vi "Historical Trend.vi"(8 "error in (no error)":errorcluster, 10 "Subview Stop Event":refnum<user-event>, 11 "Subsystem URL":refnum<k21>="\\\\localhost\\SCADA Server\\Subsystem1") -> ()   [LabVIEW 2024]
doc: "Displays the historical data for the specified subsystems. This VI is a subview of the Detailed View."
uses:
  Controls/Client/Historical Trend - Data.ctl
  Controls/Client/Historical Data.ctl
  Controls/Client/Initialization Status.ctl
  Globals/Global - Client.vi
  Shared/User Event - Stop.lvlib
panel:
  out "error out":errorcluster
  in  "End Time Stamp":timestamp=timestamp(-9593251200 s since 1904-01-01) format="%<%X\n%x>T"
  in  "Start Time Stamp":timestamp=timestamp(-9593251200 s since 1904-01-01) format="%<%X\n%x>T"
  out "Historical Data Graph":T1(graph)
  in  "Stop":bool
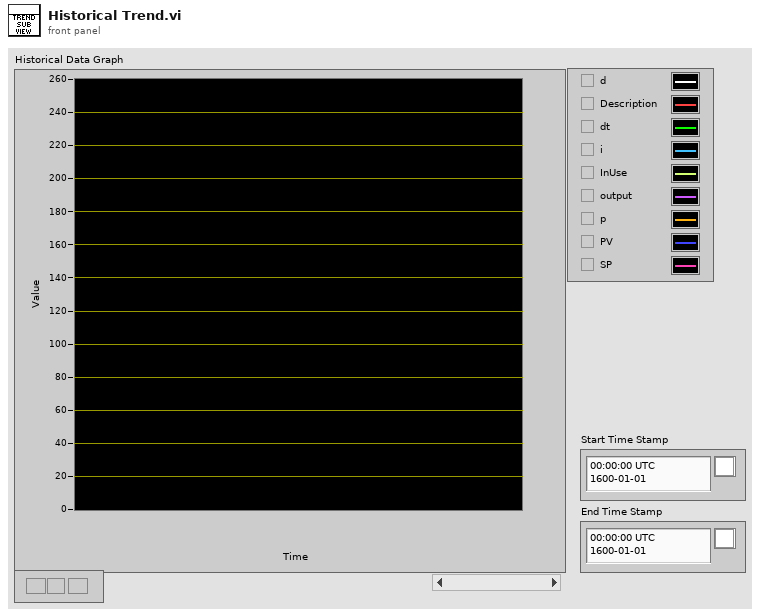
[diagram p1: front panel]
types:
  T1 = cluster{"timestamps":timestamp[], "data":dbl[]}[]
  T2 = typedef "Historical Trend - Data.ctl" = cluster{"Filtered Names":string[], "Variable URLs":refnum<k21>[], "Historical Data":T3[], "Subsystem URL":refnum<k21>, "Subview Stop Event":refnum<user-event>, "Initialization Status":T4}
  T3 = typedef "Historical Data.ctl" = cluster{"timestamps":timestamp[], "data":dbl[]}
  T4 = typedef "Initialization Status.ctl" = enum16{"Initializing", "Initialized"}
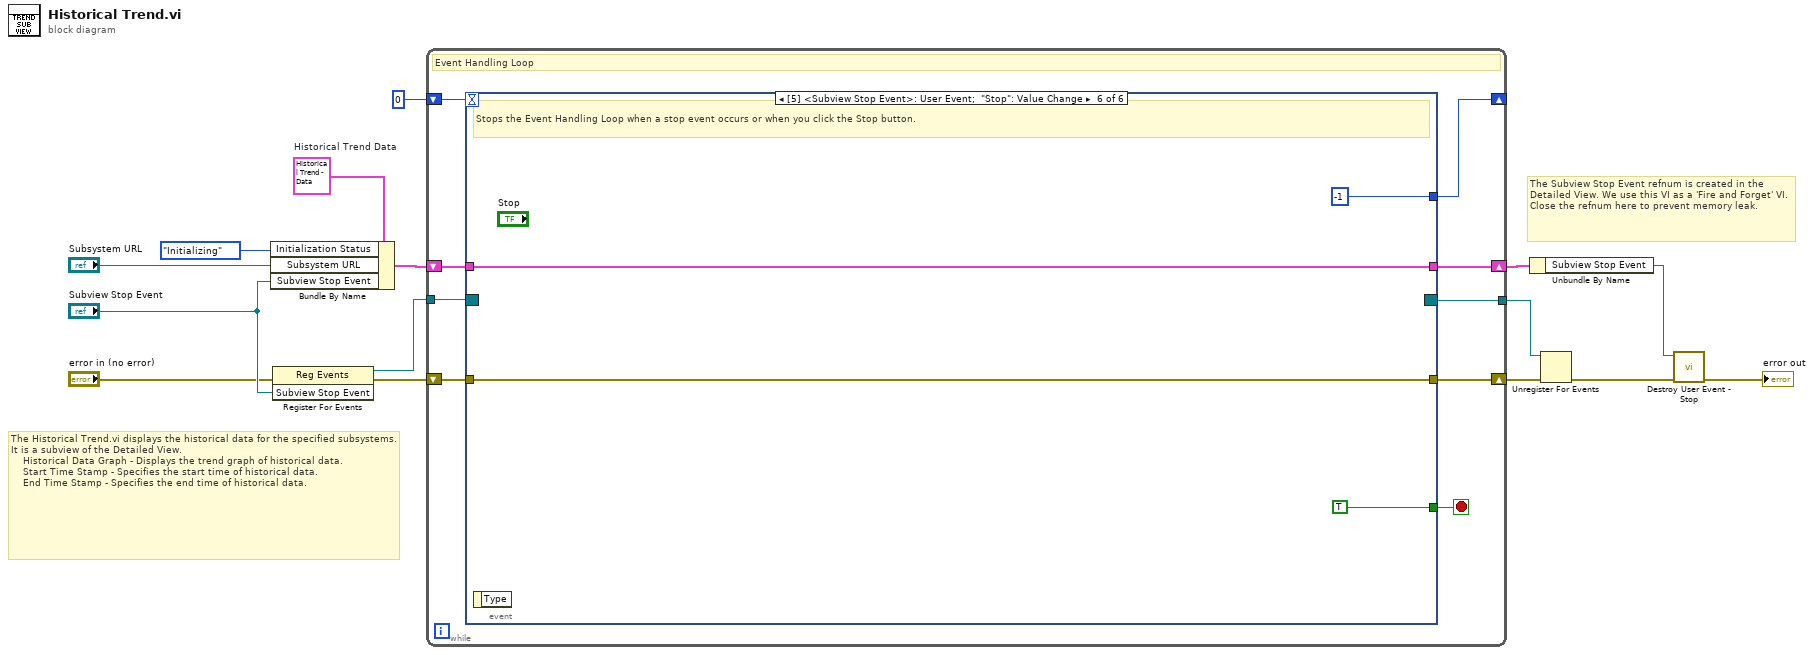
[diagram p0: block diagram]
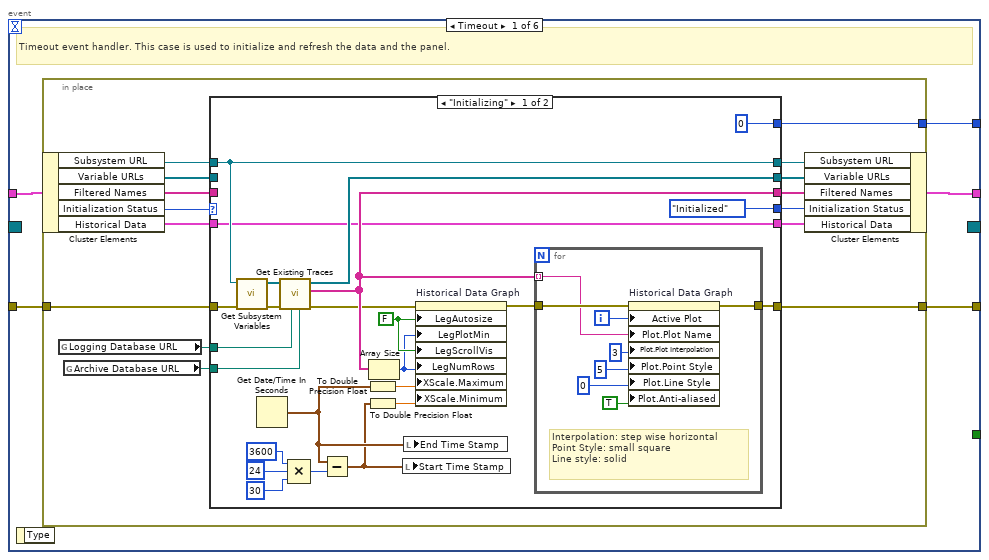
[diagram p2: hidden frame]
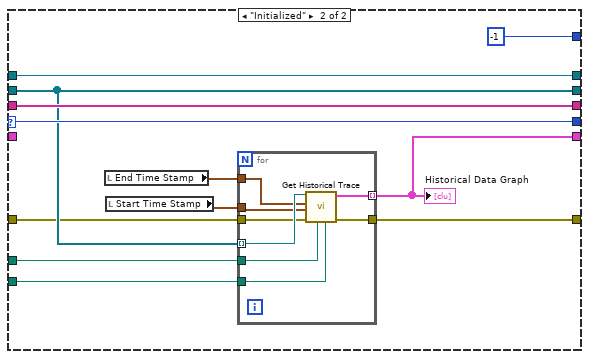
[diagram p3: hidden frame]
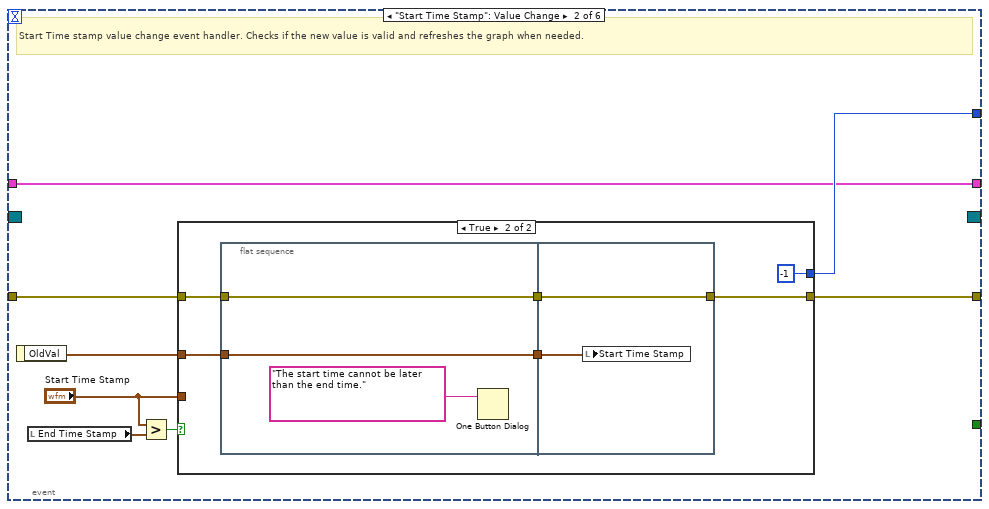
[diagram p4: hidden frame]
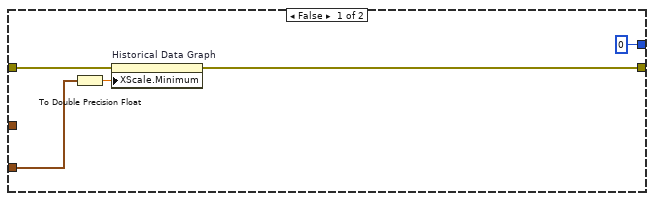
[diagram p5: hidden frame]
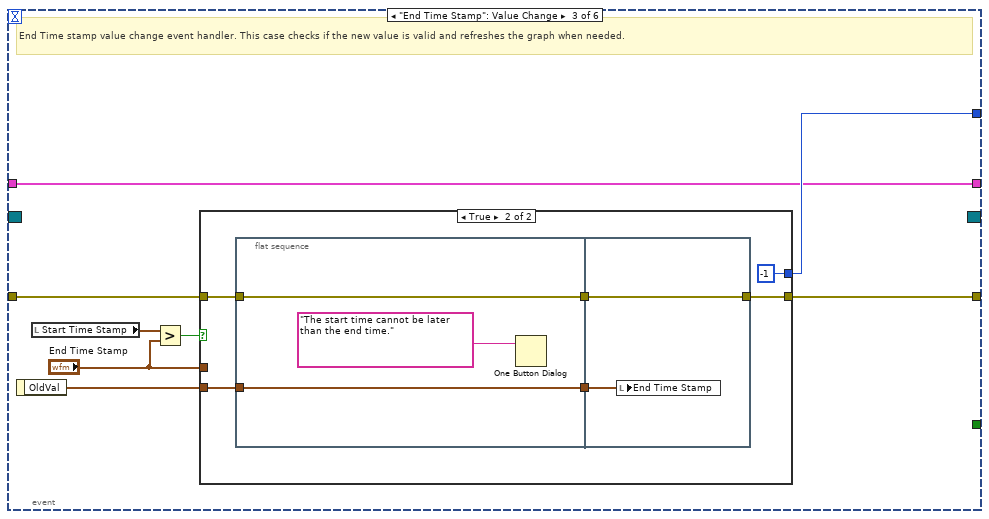
[diagram p6: hidden frame]
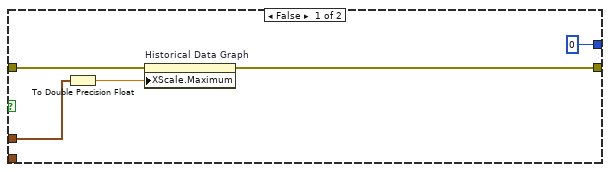
[diagram p7: hidden frame]
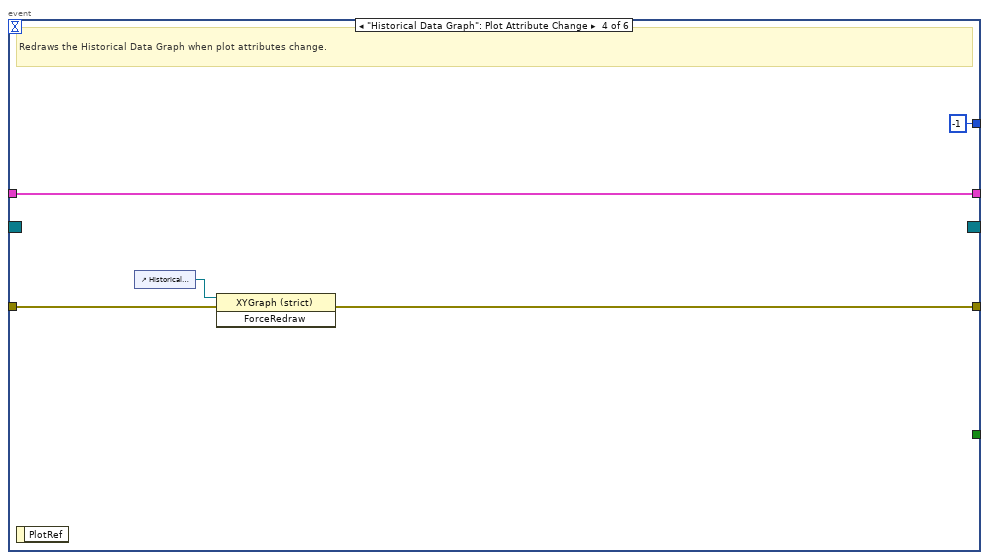
[diagram p8: hidden frame]
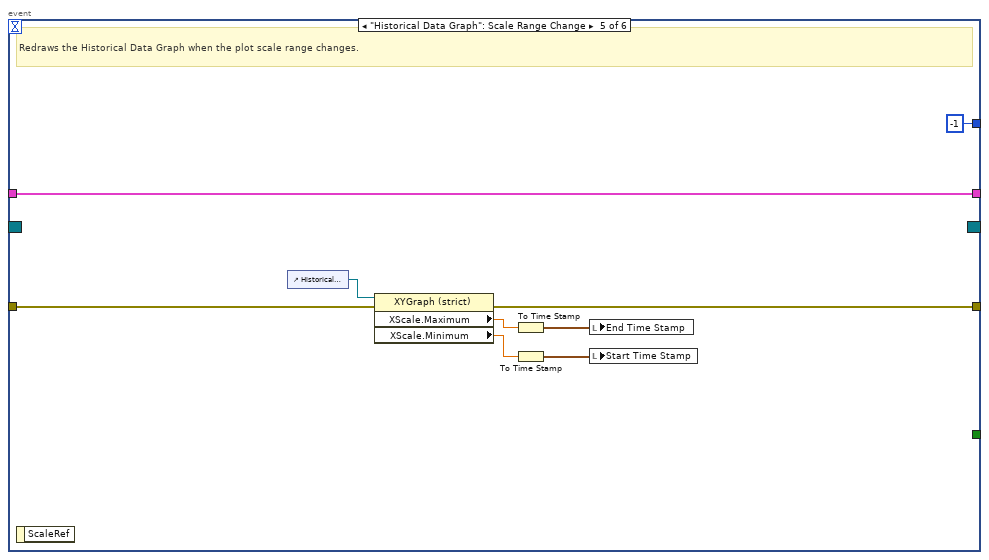
[diagram p9: hidden frame]
diagram:
  w13 = T2 {"Filtered Names"=[], "Variable URLs"=[], "Historical Data"=[], "Subsystem URL"="", "Subview Stop Event"=refnum, "Initialization Status"=enum."Initializing"}  # Historical Trend Data
  # "The Subview Stop Event refnum is created in the Detailed View. We use this VI as a 'Fire and Forget' VI. Close the refnum here to prevent memory leak."
  # "The Historical Trend.vi displays the historical data for the specified subsystems. It is a subview of the Detailed View.\n    Historical Data Graph - Displays the trend graph of historical data.\n    Start Time Stamp - Specifies the start time of historical data.\n    End Time Stamp - Specifies the end time of historical data."
  n1 = Bundle By Name(cluster=w13, "Initialization Status"=enum16{"Initializing", "Initialized"}."Initializing", "Subsystem URL"="Subsystem URL", "Subview Stop Event"="Subview Stop Event") -> (w2:T2)
  n2 = register-events(error in="error in (no error)", "Subview Stop Event") -> (reference out=w15:refnum<event-registration>, error out=w4:errorcluster)  [unwired: 1 in]
  n3 = while {
    shift-right: [w21] -> w9
    shift-left: w4 -> [w22]
    tunnel: w15 -> [w23]
    shift-right: [w19] -> _
    shift-left: 0 -> [w20]
    shift-right: [w17] -> w11
    shift-left: w2 -> [w18]
    tunnel: [w16] -> w7
    stop <- w24 stop-if-true
    # "Event Handling Loop"
    n4 = event shown="[5] <Subview Stop Event>: User Event;  \"Stop\": Value Change" {
      selector: w23 -> [_ _ _ _ _ _]
      dyn-events: [_ _ _ _ _ _] -> w16
      timeout: w20 -> [_ _ _ _ _ _]
      tunnel: [_ _ _ _ _ TRUE] -> w24
      tunnel: w22 -> [w29 w99 w123 w147 w152 w159]
      tunnel: [w27 w103 w126 w145 w151 w159] -> w21
      tunnel: [w25 w101 w125 -1 -1 -1] -> w19
      tunnel: w18 -> [w28 w100 w124 w148 w158 w160]
      tunnel: [w26 w100 w124 w148 w158 w160] -> w17
      event Timeout {
        # "Timeout event handler. This case is used to initialize and refresh the data and the panel."
        n5 = event-data() -> ()  [unwired: 1 in, 1 out]
        n6 = in-place {
          in-place-border: w29 -> [w39]
          in-place-border: [w36] -> w27
          in-place-border: [w30] -> w25
          n7 = in-place-cluster #1(w28) -> ("Subsystem URL"=w41:refnum<k21>, "Variable URLs"=w42:refnum<k21>[], "Filtered Names"=w43:string[], "Initialization Status"=w33:T4, "Historical Data"=w32:T3[])
          n8 = global read "Global - Client.vi" "Logging Database URL"() -> (w35:path)
          n9 = global read "Global - Client.vi" "Archive Database URL"() -> (w34:path)
          n10 = case shown="\"Initializing\"" w33 {
            selector: w33 -> [_ w88]
            tunnel: [enum16{"Initializing", "Initialized"}."Initialized" ("Initialization Status") w88] -> w44
            tunnel: w43 -> [_ w86]
            tunnel: w42 -> [_ w85]
            tunnel: w41 -> [w59 w87]
            tunnel: [w59 w87] -> w40
            tunnel: w39 -> [w61 w77]
            tunnel: [w57 w86] -> w38
            tunnel: [w60 w85] -> w37
            tunnel: [w56 w78] -> w36
            tunnel: w35 -> [w54 w84]
            tunnel: w34 -> [w53 w83]
            tunnel: w32 -> [w52 _]
            tunnel: [w52 w82] -> w31
            tunnel: [0 -1] -> w30
            frame "Initializing" {
              w50 = FALSE ("Legend:Autosize")
              n11 = call "Get Subsystem Variables.vi"("error in (no error)"=w61, "Subsystem URL"=w59) -> ("error out"=w63:errorcluster, "Variable URLs"=w62:refnum<k21>[])  [unwired: 6 in, 2 out]
              n12 = Get Date/Time In Seconds() -> (seconds since 1Jan1904=w48:timestamp)
              n13 = call "Get Existing Traces.vi"("Archive Database"=w53, "Logging Database"=w54, "error in (no error)"=w63, "Shared Variable URLs"=w62) -> ("error out"=w55:errorcluster, "Filtered Names"=w57:string[], "Filtered Shared Variable URLs"=w60:refnum<k21>[])  [unwired: 5 in]
              n14 = Compound Arithmetic op=MULTIPLY(3600 ("Offset(Seconds)"), 24 ("Offset(Seconds)"), 30 ("Offset(Seconds)")) -> (w68:i32)
              n15 = Subtract(x=w48, y=w68) -> (x-y=w45:timestamp)
              n16 = To Double Precision Float(number=w48) -> (double precision float=w47:dbl)
              n17 = To Double Precision Float(number=w45) -> (double precision float=w46:dbl)
              n18 = Array Size(array=w57) -> (size(s)=w49:i32)
              n19 = local write "Start Time Stamp"(w45) -> ()
              n20 = local write "End Time Stamp"(w48) -> ()
              n21 = property on="Historical Data Graph" class="XYGraph (strict)"(error in=w55, "LegAutosize"=w50, "LegPlotMin"=w49, "LegScrollVis"=w50, "LegNumRows"=w49, "XScale.Maximum"=w47, "XScale.Minimum"=w46) -> (error out=w58:errorcluster)  [unwired: 1 in, 1 out]
              n22 = for {
                tunnel: w57 -> [w73] mode=indexing
                tunnel: w58 -> [w76]
                tunnel: [w75] -> w56
                i -> [w74]
                # "Interpolation: step wise horizontal\nPoint Style: small square\nLine style: solid"
                n23 = property on="Historical Data Graph" class="XYGraph (strict)"(error in=w76, "Active Plot"=w74, "Plot.Plot Name"=w73, "Plot.Plot Interpolation"=u8 3, "Plot.Point Style"=u8 5 ("Plot.Plot Interpolation"), "Plot.Line Style"=u8 0, "Plot.Anti-aliased"=TRUE) -> (error out=w75:errorcluster)  [unwired: 1 in, 1 out]
              }
            }
            frame "Initialized" {
              n24 = local read "End Time Stamp"() -> (w81:timestamp)
              n25 = local read "Start Time Stamp"() -> (w80:timestamp)
              n26 = for {
                tunnel: w85 -> [w96] mode=indexing
                tunnel: [w95] -> w82 mode=indexing
                tunnel: w84 -> [w92]
                tunnel: w83 -> [w91]
                tunnel: w81 -> [w90]
                tunnel: w80 -> [w89]
                tunnel: w77 -> [w94]
                tunnel: [w93] -> w78
                n27 = call "Get Historical Trace.vi"("Archive Database"=w91, "Logging Database"=w92, "error in (no error)"=w94, "Start Time Stamp"=w89, "End Time Stamp"=w90, "Trace Name"=w96) -> ("error out"=w93:errorcluster, "Historical Data"=w95:T3)  [unwired: 4 in]
              }
              "Historical Data Graph" <- w82
            }
          }
          n28 = in-place-cluster #1("Subsystem URL"=w40, "Variable URLs"=w37, "Filtered Names"=w38, "Initialization Status"=w44, "Historical Data"=w31) -> (w26:T2)
        }
      }
      event "Start Time Stamp": Value Change {
        # "Start Time stamp value change event handler. Checks if the new value is valid and refreshes the graph when needed."
        n29 = event-data() -> ("OldVal"=w102:timestamp)  [unwired: 1 in]
        n30 = local read "End Time Stamp"() -> (w98:timestamp)
        n31 = Greater?(x="Start Time Stamp", y=w98) -> (0:w104:bool)
        n32 = case shown="True" w104 {
          tunnel: w102 -> [_ w115]
          tunnel: w99 -> [w108 w114]
          tunnel: [w107 w113] -> w103
          tunnel: [0 -1] -> w101
          tunnel: "Start Time Stamp" -> [w106 _]
          frame False {
            n33 = To Double Precision Float(number=w106) -> (double precision float=w105:dbl)
            n34 = property on="Historical Data Graph" class="XYGraph (strict)"(error in=w108, "XScale.Minimum"=w105) -> (error out=w107:errorcluster)  [unwired: 1 in, 1 out]
          }
          frame True {
            n35 = flat-sequence {
              tunnel: w114 -> [w117]
              tunnel: w115 -> [w118]
              tunnel: [w118] -> w111
              tunnel: [w117] -> w110
              tunnel: [w120] -> w113
              tunnel: w111 -> [w119]
              tunnel: w110 -> [w120]
              frame #0 {
                n36 = One Button Dialog(message="The start time cannot be later  than the end time.") -> ()  [unwired: 1 in, 1 out]
              }
              frame #1 {
                n37 = local write "Start Time Stamp"(w119) -> ()
              }
            }
          }
        }
      }
      event "End Time Stamp": Value Change {
        # "End Time stamp value change event handler. This case checks if the new value is valid and refreshes the graph when needed."
        n38 = event-data() -> ("OldVal"=w127:timestamp)  [unwired: 1 in]
        n39 = local read "Start Time Stamp"() -> (w122:timestamp)
        n40 = Greater?(x=w122, y="End Time Stamp") -> (0:w128:bool)
        n41 = case shown="True" w128 {
          tunnel: w127 -> [_ w139]
          tunnel: w123 -> [w132 w138]
          tunnel: [w131 w137] -> w126
          tunnel: [0 -1] -> w125
          tunnel: "End Time Stamp" -> [w129 _]
          frame False {
            n42 = To Double Precision Float(number=w129) -> (double precision float=w130:dbl)
            n43 = property on="Historical Data Graph" class="XYGraph (strict)"(error in=w132, "XScale.Maximum"=w130) -> (error out=w131:errorcluster)  [unwired: 1 in, 1 out]
          }
          frame True {
            n44 = flat-sequence {
              tunnel: w138 -> [w141]
              tunnel: w139 -> [w142]
              tunnel: [w142] -> w135
              tunnel: [w141] -> w134
              tunnel: [w144] -> w137
              tunnel: w135 -> [w143]
              tunnel: w134 -> [w144]
              frame #0 {
                n45 = One Button Dialog(message="The start time cannot be later  than the end time.") -> ()  [unwired: 1 in, 1 out]
              }
              frame #1 {
                n46 = local write "End Time Stamp"(w143) -> ()
              }
            }
          }
        }
      }
      event "Historical Data Graph": Plot Attribute Change {
        # "Redraws the Historical Data Graph when plot attributes change."
        n47 = event-data() -> ()  [unwired: 1 in, 1 out]
        n48 = control-ref of="Historical Data Graph"() -> (w146:refnum<vi>)
        n49 = invoke class="XYGraph (strict)" method="ForceRedraw"(reference=w146, error in=w147) -> (error out=w145:errorcluster)  [unwired: 1 in, 2 out]
      }
      event "Historical Data Graph": Scale Range Change {
        # "Redraws the Historical Data Graph when the plot scale range changes."
        n50 = event-data() -> ()  [unwired: 1 in, 1 out]
        n51 = control-ref of="Historical Data Graph"() -> (w153:refnum<vi>)
        n52 = property class="XYGraph (strict)"(reference=w153, error in=w152) -> (error out=w151:errorcluster, "XScale.Maximum"=w156:dbl, "XScale.Minimum"=w157:dbl)  [unwired: 1 out]
        n53 = To Time Stamp(1:w156) -> (0:w155:timestamp)
        n54 = To Time Stamp(1:w157) -> (0:w154:timestamp)
        n55 = local write "End Time Stamp"(w155) -> ()
        n56 = local write "Start Time Stamp"(w154) -> ()
      }
      event User Event; "Stop": Value Change {
        # "Stops the Event Handling Loop when a stop event occurs or when you click the Stop button."
        n57 = event-data() -> ()  [unwired: 1 in, 1 out]
      }
    }
  }
  n58 = Unbundle By Name(w11) -> ("Subview Stop Event"=w10:refnum<user-event>)
  n59 = Unregister For Events(event registration refnum=w7, error in=w9) -> (error out=w8:errorcluster)
  n60 = call "Destroy User Event - Stop.vi"("error in (no error)"=w8, "User Event - Stop"=w10) -> ("error out"=→"error out":errorcluster)  [unwired: 9 in]
